vi "Get Frame Count.vi"(8 "error in (no error)":errorcluster, 11 "Camera in":refnum<class "Camera.lvclass">) -> (0 "error out":errorcluster, 2 "Frame Count":i64, 3 "Camera":refnum<class "Camera.lvclass">)   [LabVIEW 2020, in "Camera.lvclass"]
doc: "Set the Number of Frames to capture during Fixed Frame Acqusition streaming operation."
uses:
  Camera.lvclass
  Camera.lvclass/Camera.ctl
  Check Not Disconnected.vi
  <vilib>/Utility/error.llb/Error Cluster From Error Code.vi
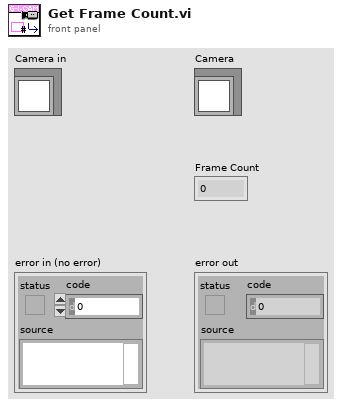
[diagram p1: front panel]
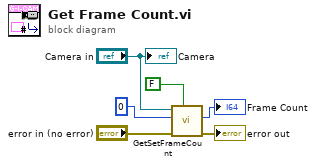
[diagram p0: block diagram]
diagram:
  n1 = call "GetSetFrameCount.vi"("Set"=FALSE, "error in (no error)"="error in (no error)", "Frame Count"=i64 0, "Camera in"="Camera in") -> ("error out"=→"error out":errorcluster, "Frame Count"=→"Frame Count":i64)  [unwired: 6 in]
  "Camera" <- "Camera in"
